vi "Configure.vi"(8 "error in (no error)":errorcluster, 11 "AM-AM in":refnum<class "AM-AM.lvclass">) -> (0 "error out":errorcluster, 3 "AM-AM out":refnum<class "AM-AM.lvclass">)   [LabVIEW 2020, in "AM-AM.lvclass"]
doc: "Configure the measurements paramaters to sweep.\nThis should be a pop up interface invoked by the configure test button on the main panel."
uses:
  AM-AM.lvclass
  Controls/Loop order.ctl
  AM-AM.lvclass/AM-AM.ctl
  Controls/Config info.ctl
panel:
  in  "Power Window":dbl format="%#_6p"
  in  "Loop order":T1
  in  "OK Button":bool
  in  "Average On":bool
  in  "Number of Averages":dbl
  in  "VBW":dbl format="%#_6p"
  in  "RBW":dbl format="%#_6p"
  in  "Power":enum32{"From To", "Array"}(tab)
  in  "Power Cluster":cluster{"From":dbl, "To":dbl, "Step":dbl}
  in  "Power Array":dbl[](array[numeric]) format="%#_6p"
  in  "Frequency":enum32{"From To", "Array"}(tab)
  in  "Frequency Cluster":cluster{"From":dbl, "To":dbl, "Step":dbl}
  in  "Frequency Array":dbl[](array[numeric]) format="%#_6p"
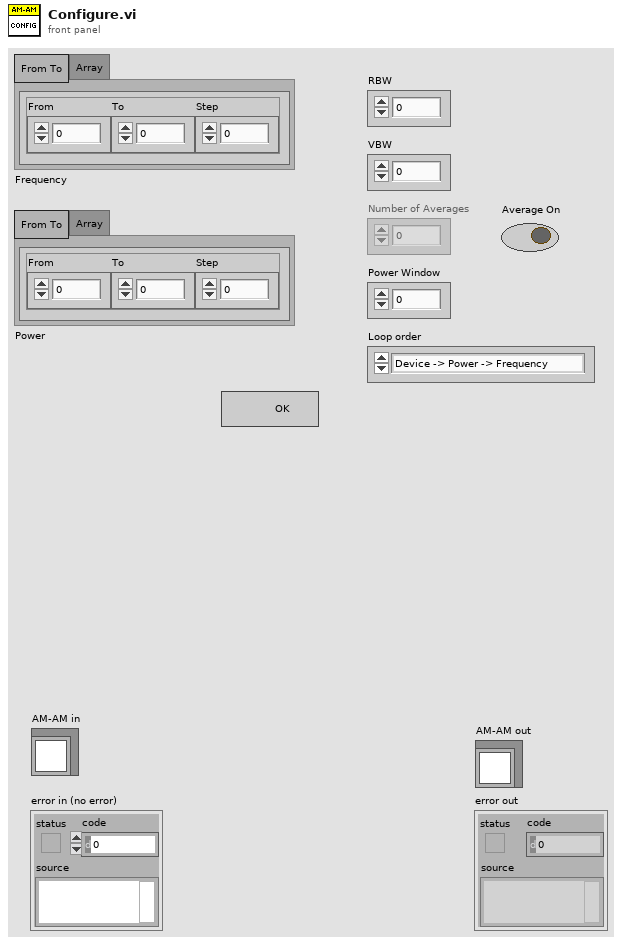
[diagram p1: front panel]
types:
  T1 = typedef "AM-AM.lvclass/Loop order.ctl" = enum16{"Device -> Power -> Frequency", "Device -> Frequency -> Power"}
  T2 = enum8{"Enabled", "Disabled", "Disabled and Grayed Out"}
  T3 = typedef "AM-AM.lvclass/Config info.ctl" = cluster{"RBW":dbl, "VBW ":dbl, "Number of Averages":dbl, "Average On":bool, "Power":cluster{"Cluster ":cluster{"From":dbl, "To":dbl, "Step":dbl}, "Array":dbl[], "Use Array":bool}, "Frequency":cluster{"Cluster ":cluster{"From":dbl, "To":dbl, "Step":dbl}, "Array":dbl[], "Use Array":bool}, "Loop order":T1, "Power Window":dbl}
  T4 = cluster{"Cluster ":cluster{"From":dbl, "To":dbl, "Step":dbl}, "Array":dbl[], "Use Array":bool}
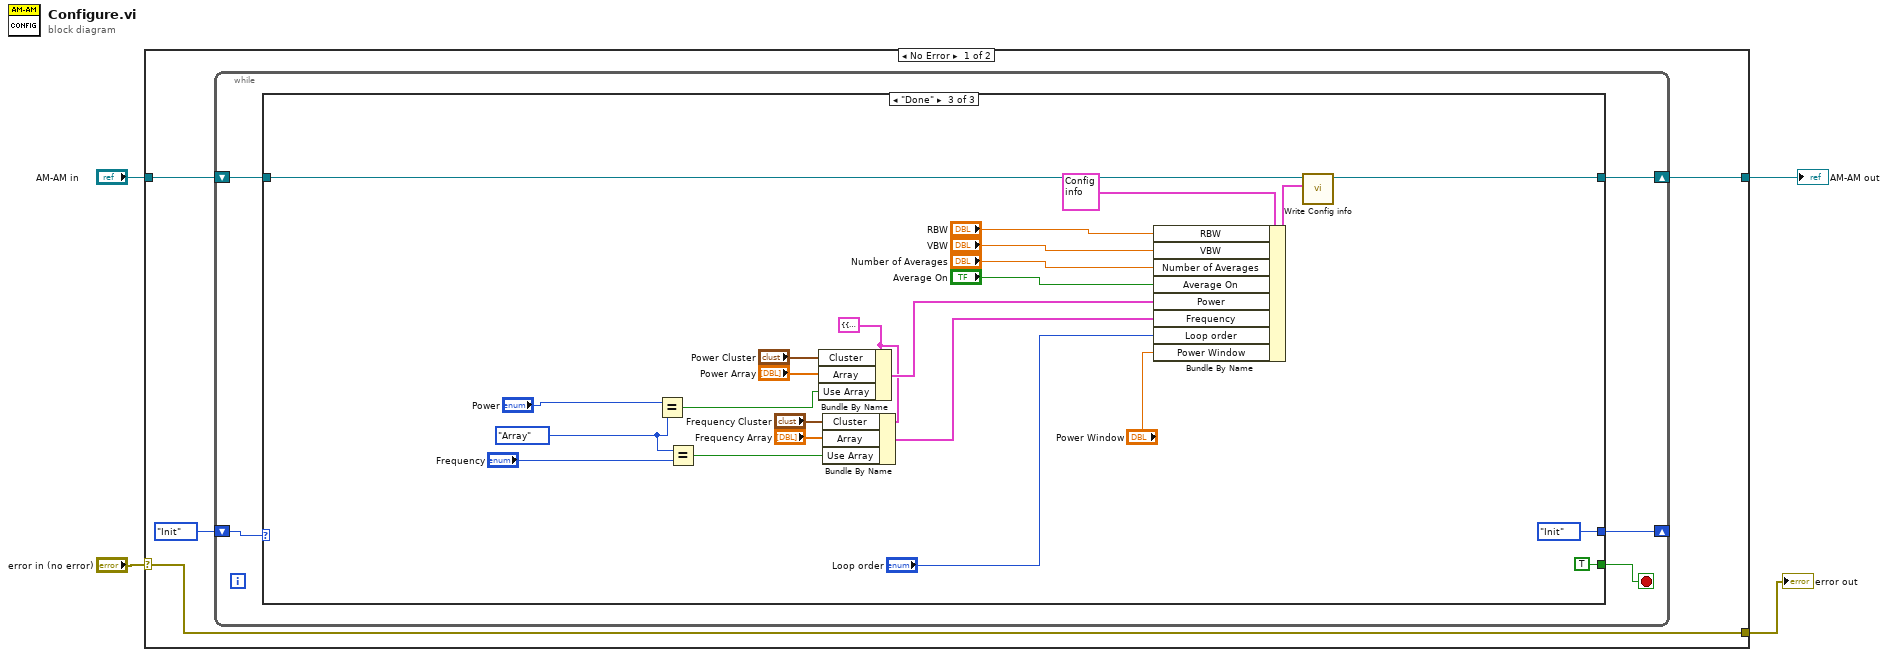
[diagram p0: block diagram]
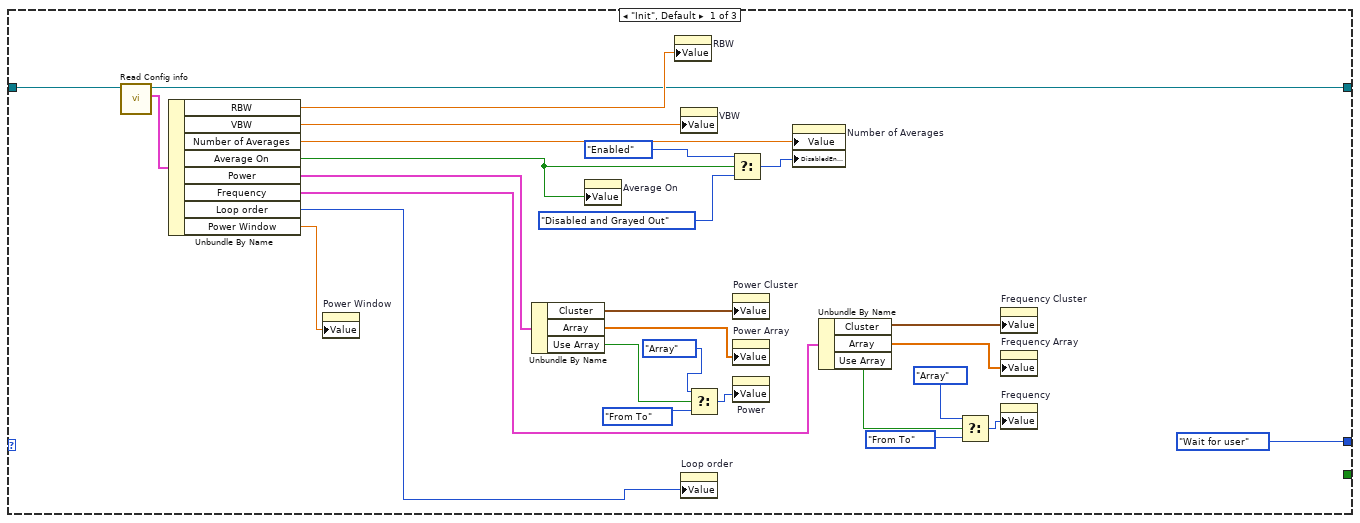
[diagram p2: hidden frame]
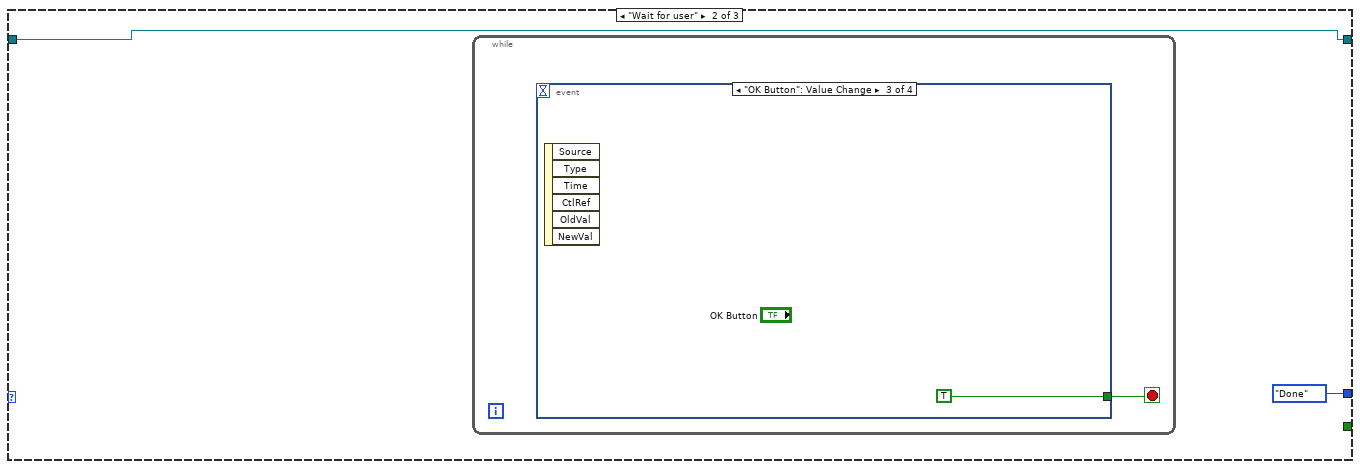
[diagram p3: hidden frame]
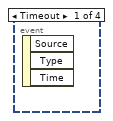
[diagram p4: hidden frame]
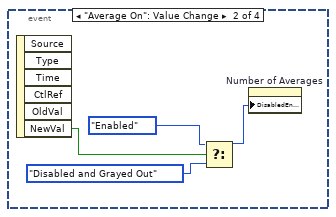
[diagram p5: hidden frame]
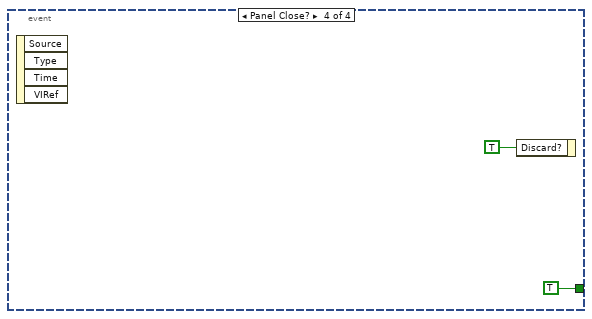
[diagram p6: hidden frame]
diagram:
  n1 = case shown="No Error" "error in (no error)" {
    selector: "error in (no error)" -> [w5 w75]
    tunnel: "AM-AM in" -> [w8 w76]
    tunnel: [w7 w76] -> w2
    tunnel: [w5 w75] -> w1
    frame No Error {
      n2 = while {
        shift-right: [w12] -> w7
        shift-left: w8 -> [w13]
        shift-right: [w10] -> _
        shift-left: enum16{"Init", "Wait for user", "Done"}."Init" -> [w11]
        stop <- w9 stop-if-true
        n3 = case shown="\"Done\"" w11 {
          tunnel: w13 -> [w40 w42 w71]
          tunnel: [w18 w42 w72] -> w12
          tunnel: [enum16{"Init", "Wait for user", "Done"}."Wait for user" enum16{"Init", "Wait for user", "Done"}."Done" enum16{"Init", "Wait for user", "Done"}."Init"] -> w10
          tunnel: [_ _ TRUE] -> w9
          frame "Init", Default {
            n4 = call "Read Config info.vi"("AM-AM in"=w40) -> ("Config info"=w39:T3, "AM-AM out"=w18:refnum<class "AM-AM.lvclass">)  [unwired: 9 in]
            n5 = Unbundle By Name(w39) -> ("RBW"=w38:dbl, "VBW"=w37:dbl, "Number of Averages"=w15:dbl, "Average On"=w33:bool, "Power"=w32:T4, "Frequency"=w25:T4, "Loop order"=w16:T1, "Power Window"=w14:dbl)
            n6 = property on="Power Window" class="DigNum (strict)"("Value"=w14) -> ()  [unwired: 2 in, 2 out]
            n7 = Unbundle By Name(w32) -> ("Cluster"=w31:cluster{"From":dbl, "To":dbl, "Step":dbl}, "Array"=w30:dbl[], "Use Array"=w27:bool)
            n8 = property on="Average On" class="Bool (strict)"("Value"=w33) -> ()  [unwired: 2 in, 2 out]
            n9 = property on="RBW" class="DigNum (strict)"("Value"=w38) -> ()  [unwired: 2 in, 2 out]
            n10 = property on="VBW" class="DigNum (strict)"("Value"=w37) -> ()  [unwired: 2 in, 2 out]
            n11 = property on="Loop order" class="Enum (strict)"("Value"=w16) -> ()  [unwired: 2 in, 2 out]
            n12 = Select(t=enum32{"From To", "Array"}."Array" ("Power"), s=w27, f=enum32{"From To", "Array"}."From To") -> (s? t:f=w29:enum32{"From To", "Array"})
            n13 = Select(t=T2."Enabled" ("Disabled"), s=w33, f=T2."Disabled and Grayed Out") -> (s? t:f=w35:T2)
            n14 = property on="Power Cluster" class="Clust (strict)"("Value"=w31) -> ()  [unwired: 2 in, 2 out]
            n15 = property on="Power Array" class="Arr (strict)"("Value"=w30) -> ()  [unwired: 2 in, 2 out]
            n16 = property on="Power" class="TabCtl (strict)"("Value"=w29) -> ()  [unwired: 2 in, 2 out]
            n17 = property on="Number of Averages" class="DigNum (strict)"("Value"=w15, "DisabledEnum"=w35) -> ()  [unwired: 2 in, 2 out]
            n18 = Unbundle By Name(w25) -> ("Cluster"=w24:cluster{"From":dbl, "To":dbl, "Step":dbl}, "Array"=w23:dbl[], "Use Array"=w19:bool)
            n19 = Select(t=enum32{"From To", "Array"}."Array" ("Power"), s=w19, f=enum32{"From To", "Array"}."From To") -> (s? t:f=w21:enum32{"From To", "Array"})
            n20 = property on="Frequency Cluster" class="Clust (strict)"("Value"=w24) -> ()  [unwired: 2 in, 2 out]
            n21 = property on="Frequency Array" class="Arr (strict)"("Value"=w23) -> ()  [unwired: 2 in, 2 out]
            n22 = property on="Frequency" class="TabCtl (strict)"("Value"=w21) -> ()  [unwired: 2 in, 2 out]
          }
          frame "Wait for user" {
            n23 = while {
              stop <- w43 stop-if-true
              n24 = event shown="[2] \"OK Button\": Value Change" {
                selector: _ -> [_ _ _ _]
                dyn-events: _ -> [_ _ _ _]
                timeout: _ -> [_ _ _ _]
                tunnel: [_ _ TRUE TRUE] -> w43
                event Timeout {
                  n25 = event-data() -> ()  [unwired: 1 in, 3 out]
                }
                event "Average On": Value Change {
                  n26 = event-data() -> ("NewVal"=w47:bool)  [unwired: 1 in, 5 out]
                  n27 = Select(t=T2."Enabled" ("Disabled"), s=w47, f=T2."Disabled and Grayed Out" ("Disabled")) -> (s? t:f=w46:T2)
                  n28 = property on="Number of Averages" class="DigNum (strict)"("DisabledEnum"=w46) -> ()  [unwired: 2 in, 2 out]
                }
                event "OK Button": Value Change {
                  n29 = event-data() -> ()  [unwired: 1 in, 6 out]
                }
                event Panel Close? {
                  n30 = event-data() -> ()  [unwired: 1 in, 4 out]
                  n31 = event-data("Discard?"=TRUE) -> ()  [unwired: 1 in, 1 out]
                }
              }
            }
          }
          frame "Done" {
            w56 = enum32{"From To", "Array"}."Array" ("y")
            w62 = T4 {"Cluster "={"From"=0.0, "To"=0.0, "Step"=0.0}, "Array"=[], "Use Array"=FALSE} ("Power")
            n32 = Equal?(x="Power", y=w56) -> (x = y?=w58:bool)
            n33 = Equal?(x=w56, y="Frequency") -> (x = y?=w55:bool)
            n34 = Bundle By Name(cluster=w62, "Cluster"="Power Cluster", "Array"="Power Array", "Use Array"=w58) -> (w63:T4)
            n35 = Bundle By Name(cluster=w62, "Cluster"="Frequency Cluster", "Array"="Frequency Array", "Use Array"=w55) -> (w61:T4)
            n36 = Bundle By Name(cluster=T3 {"RBW"=0.0, "VBW "=0.0, "Number of Averages"=0.0, "Average On"=FALSE, "Power"={"Cluster "={"From"=0.0, "To"=0.0, "Step"=0.0}, "Array"=[], "Use Array"=FALSE}, "Frequency"={"Cluster "={"From"=0.0, "To"=0.0, "Step"=0.0}, "Array"=[], "Use Array"=FALSE}, "Loop order"=enum."Device -> Power -> Frequency", "Power Window"=0.0} ("Config info"), "RBW"="RBW", "VBW"="VBW", "Number of Averages"="Number of Averages", "Average On"="Average On", "Power"=w63, "Frequency"=w61, "Loop order"="Loop order", "Power Window"="Power Window") -> (w53:T3)
            n37 = call "Write Config info.vi"("Config info"=w53, "AM-AM in"=w71) -> ("AM-AM out"=w72:refnum<class "AM-AM.lvclass">)  [unwired: 9 in]
          }
        }
      }
    }
    frame Error {
    }
  }
  "error out" <- w1
  "AM-AM out" <- w2
